vi "U3 Hardware Counter.vi"() -> ()   [LabVIEW 2021]
panel:
  out "Counter Reads":u32[](array[numeric])
  in  "Timer/Counter Pin Offset":u8=4
  in  "Reset Counters":bool
  in  "Iteration Inverval (ms)":u32=100
  out "Iteration":i32
  in  "error in":errorcluster
  in  "Address":string="1"
  in  "FirstFound":bool=TRUE
  in  "stop":bool
  out "error out":errorcluster
  out "Error Message":string
  # "Enables both hardware counters, and reads them at the specified interval.\nSince there are no timers, the counters will be assigned to pins starting with FIO0 plus pin offset."
  # "Firmware Counter 0"
  # "Firmware Counter 1"
  # "Counter 0"
  # "Counter 1"
  # "This VI passes a timer\nbase clock constant that\nis valid for hardware V1.21.\nFor hardware V1.20 change\nLJ_tc48MHZ to LJ_tc24MHZ."
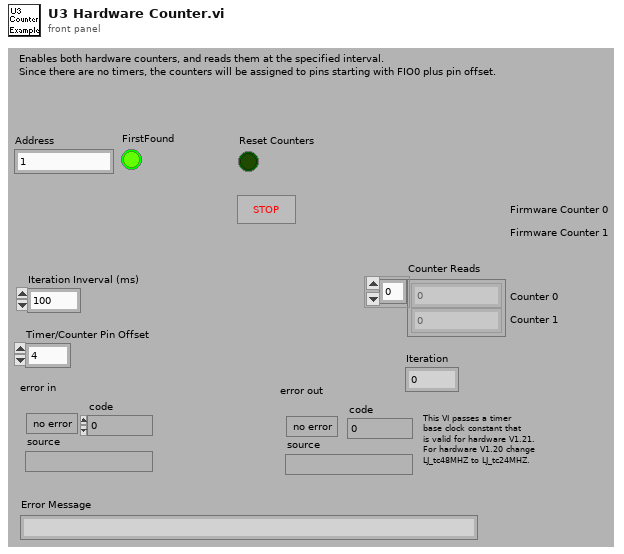
[diagram p1: front panel]
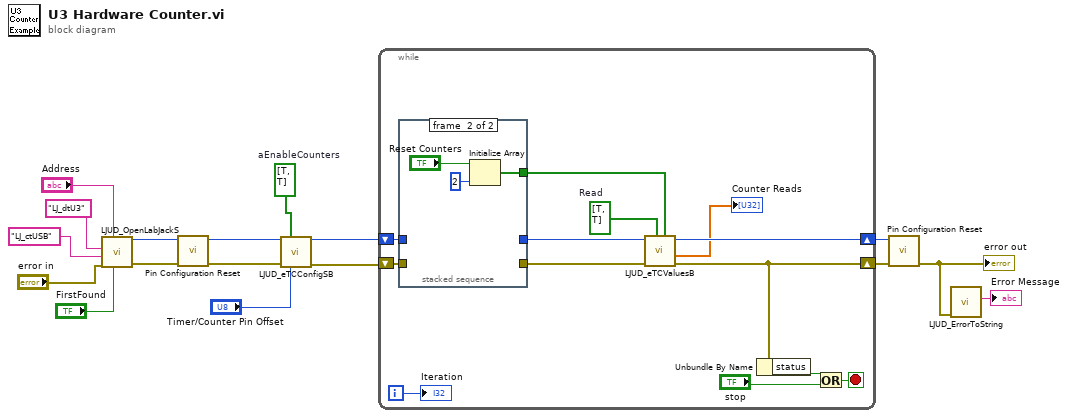
[diagram p0: block diagram]
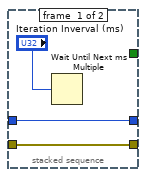
[diagram p2: hidden frame]
diagram:
  w8 = bool[] [TRUE, TRUE]  # aEnableCounters
  n1 = call "LJUD_OpenLabJackS.vi"("FirstFound"="FirstFound", "Address"="Address", "error in"="error in", "ConnectionType"="LJ_ctUSB", "DeviceType"="LJ_dtU3") -> ("error out"=w3:errorcluster, "Handle"=w4:i32)  [unwired: 4 in, 1 out]
  n2 = call "Pin Configuration Reset.vi"("error in"=w3, "Handle In"=w4) -> ("error out"=w2:errorcluster, "Handle Out"=w1:i32)  [unwired: 8 in]
  n3 = call "LJUD_eTCConfigSB.vi"("Handle In"=w1, "aEnableCounters"=w8, "error in"=w2, "TCPinOffset"="Timer/Counter Pin Offset") -> ("Handle Out"=w9:i32, "error out"=w10:errorcluster)  [unwired: 10 in]
  n4 = while {
    shift-left: w10 -> [w29]
    shift-right: [w23] -> w6
    shift-left: w9 -> [w30]
    shift-right: [w22] -> w7
    i -> [w25]
    stop <- w28 stop-if-true
    w19 = bool[] [TRUE, TRUE]  # Read
    n5 = stacked-sequence {
      tunnel: [w33 _] -> w21
      tunnel: [w32 _] -> w24
      tunnel: w30 -> [w33 _]
      tunnel: w29 -> [w32 _]
      tunnel: [_ w34] -> w20
      frame #0 {
        n6 = Wait Until Next ms Multiple(millisecond multiple="Iteration Inverval (ms)") -> ()  [unwired: 1 out]
      }
      frame #1 {
        n7 = Initialize Array("Reset Counters", 2 ("Dimension Size")) -> (w34:bool[])
      }
    }
    n8 = call "LJUD_eTCValuesB.vi"("aResetCounters"=w20, "aReadCounters"=w19, "error in"=w24, "Handle In"=w21) -> ("error out"=w23:errorcluster, "aCounterValues"=→"Counter Reads":dbl[], "Handle Out"=w22:i32)  [unwired: 4 in, 1 out]
    n9 = Unbundle By Name(w23) -> ("status"=w27:bool)
    n10 = Or(x=w27, y="stop") -> (x .or. y?=w28:bool)
    "Iteration" <- w25
  }
  n11 = call "Pin Configuration Reset.vi"("error in"=w6, "Handle In"=w7) -> ("error out"=w5:errorcluster)  [unwired: 8 in, 1 out]
  "error out" <- w5
  n12 = call "LJUD_ErrorToString.vi"("error in"=w5) -> ("String"=→"Error Message":string)  [unwired: 10 in]
